vi "TxtHeaderAdvGen.vi"(0 "VarPar":string caption="Param de Balayage Princ", 1 "NomDon":string[](array[string])=["RTêta;", "X&Y;"], 3 "2ndParam":dbl[](array[numeric]) format="%#_15e", 5 "NbCourbe":i32=1 caption="Nb de Balayage", 7 "VarPar Sec":string caption="Param de Balayage Sec", 9 "IndCourbe":i64 caption="Numéro de Balayage", 11 "error in":errorcluster, 12 "Mode":u16(ring) items=["Scan", "Log"], 14 "UnitDon":string[][](array[string])=[["(V)", "(°)"]] caption="Unités Données") -> (4 "Scan list":string[](array[string]), 10 "Entête":string, 15 "error out":errorcluster)   [LabVIEW 2010]
doc: "Ce Vi créer la ligne d'entête du fichier texte de sauvegarde à partir du nombre de courbe voulu."
panel:
  # "Chaque ligne correspond aux différentes unités de \nl'élément correspondant du tableau NomDon. Un élément \"NomDon\" peut avoir plusieurs paramètres (unités) mesurés, mais seulement le premier apparait dans la scanlist. Par contre ils apparaissent tous dans l'entête"
  # ": Chaque item correspond à un élément de plus dans la scan list"
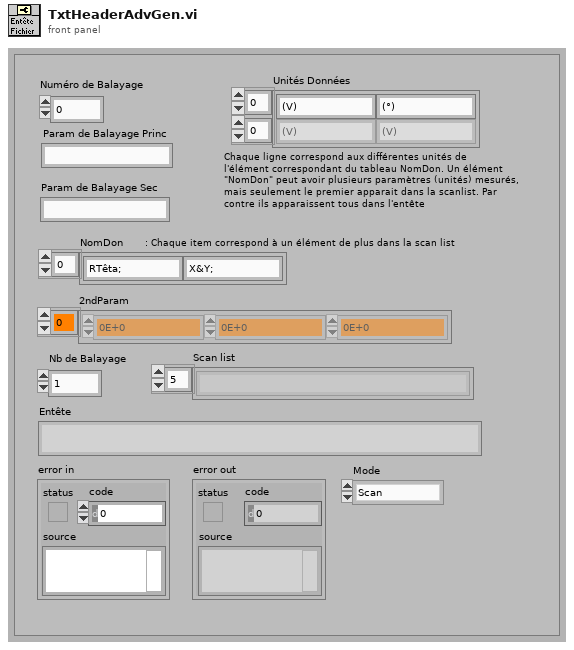
[diagram p1: front panel]
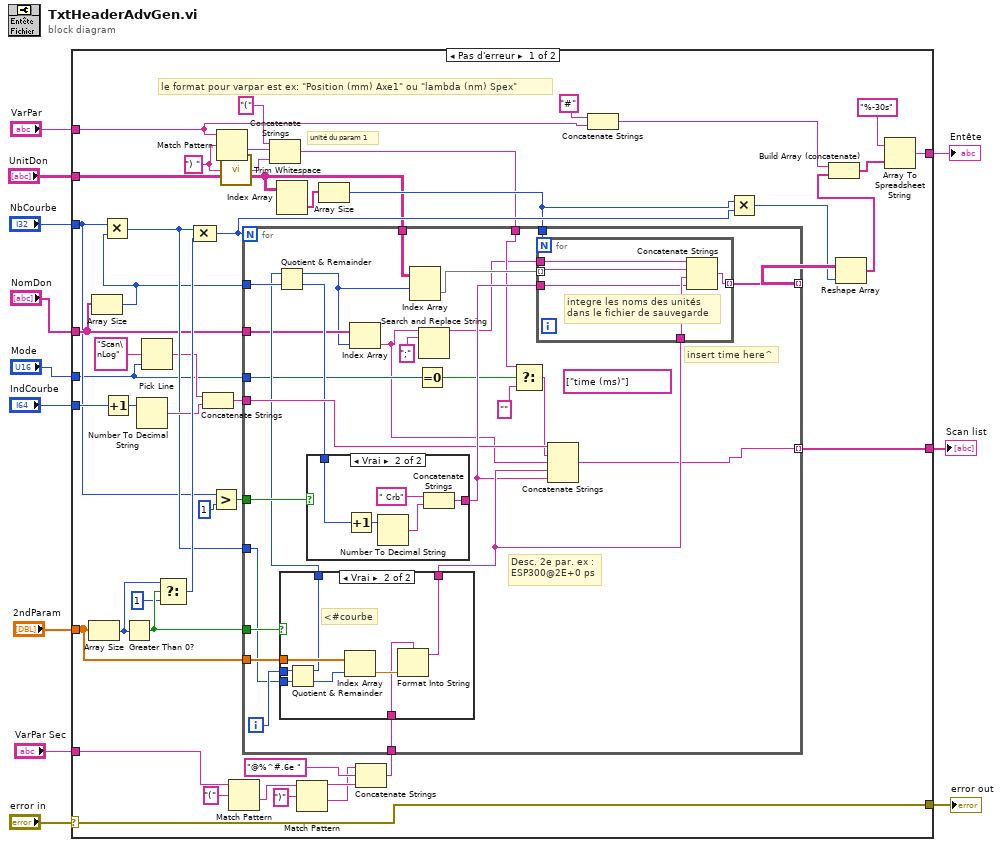
[diagram p0: block diagram]
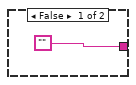
[diagram p2: hidden frame]
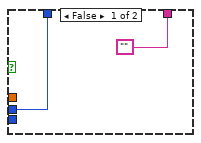
[diagram p3: hidden frame]
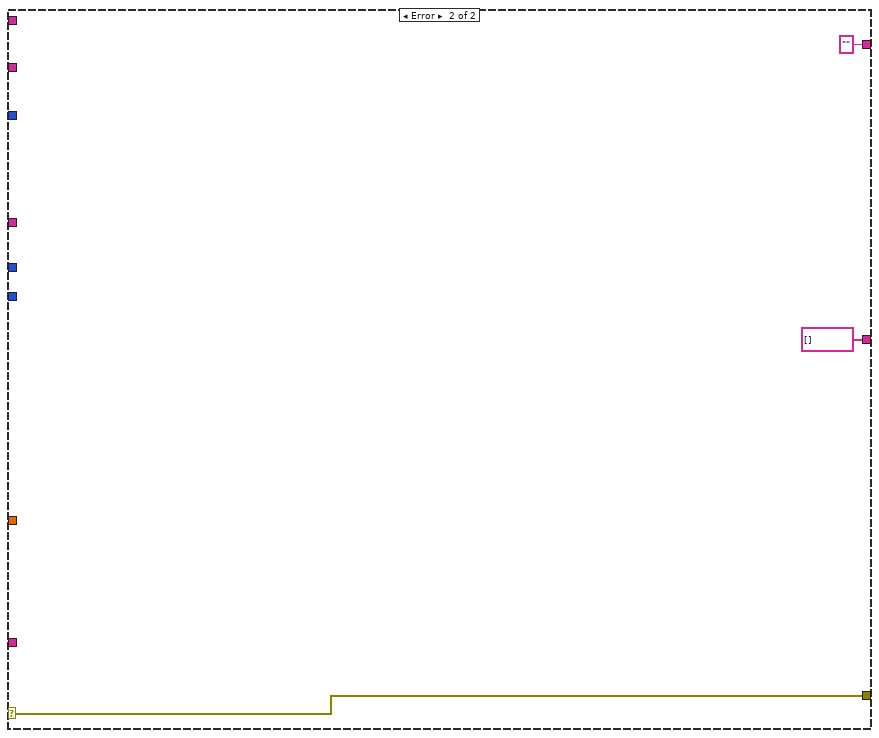
[diagram p4: hidden frame]
diagram:
  n1 = case shown="Pas d'erreur" "error in" {
    selector: "error in" -> [w56 w109]
    tunnel: [w56 w109] -> w11
    tunnel: "NbCourbe" -> [w19 _]
    tunnel: [w29 string[] []] -> w9
    tunnel: [w55 "" ("spreadsheet string")] -> w8
    tunnel: "IndCourbe" -> [w45 _]
    tunnel: "2ndParam" -> [w51 _]
    tunnel: "UnitDon" -> [w27 _]
    tunnel: "NomDon" -> [w25 _]
    tunnel: "VarPar" -> [w15 _]
    tunnel: "VarPar Sec" -> [w23 _]
    tunnel: "Mode" -> [w18 _]
    frame No Error {
      w31 = ") " ("expression régulière")
      # "le format pour varpar est ex: \"Position (mm) Axe1\" ou \"lambda (nm) Spex\""
      # "unité du param 1"
      n2 = Array Size(array=w51) -> (size(s)=w52:i32)
      n3 = Array Size(array=w25) -> (size(s)=w24:i32)
      n4 = Multiply(x=w19, y=w24) -> (x*y=w28:i32)
      n5 = Increment(x=w45) -> (x+1=w44:i64)
      n6 = Greater Than 0?(x=w52) -> (x > 0?=w54:bool)
      n7 = Number To Decimal String(number=w44) -> (decimal integer string=w39:string)  [unwired: 1 in]
      n8 = Pick Line(multi-line string="Scan\nLog", line index=w18) -> (output string=w20:string)  [unwired: 1 in]
      n9 = Select(t=w52, s=w54, f=1 ("NbCourbe")) -> (s? t:f=w46:i32)
      n10 = Compound Arithmetic op=MULTIPLY(w28, w46) -> (w41:i32)
      n11 = Concatenate Strings(w20, w39) -> (w38:string)
      n12 = Greater?(x=w19, y=1) -> (0:w43:bool)
      n13 = Match Pattern(string=w15, regular expression=w31) -> (after substring=w33:string)  [unwired: 1 in, 3 out]
      n14 = call <vilib>:"Trim Whitespace.vi"("string"=w31) -> ("trimmed string"=w30:string)  [unwired: 1 in]
      n15 = Match Pattern(string=w23, regular expression="(" ("expression régulière")) -> (after substring=w36:string)  [unwired: 1 in, 3 out]
      n16 = Concatenate Strings("(" ("expression régulière"), w33, w30) -> (w22:string)
      n17 = Index Array(array=w27) -> (element=w26:string[])  [unwired: 2 in]
      n18 = Match Pattern(string=w36, regular expression=")" ("expression régulière")) -> (before substring=w35:string, after substring=w34:string)  [unwired: 1 in, 2 out]
      n19 = Array Size(array=w26) -> (size(s)=w37:i32)
      n20 = Concatenate Strings(w34, "@%^#.6e ", w35) -> (w48:string)
      n21 = for {
        N: w41 -> [_]
        tunnel: [w63] -> w29 mode=indexing
        tunnel: w22 -> [w68]
        tunnel: w54 -> [w85]
        tunnel: w51 -> [w84]
        tunnel: w48 -> [w83]
        tunnel: w28 -> [w81]
        tunnel: w38 -> [w76]
        tunnel: [w62] -> w17 mode=indexing
        tunnel: w43 -> [w80]
        tunnel: w27 -> [w75]
        tunnel: w37 -> [w79]
        tunnel: w24 -> [w73]
        tunnel: w25 -> [w70]
        tunnel: w18 -> [w67]
        i -> [w82]
        (unwired) string[] ["time (ms)"] ("tableau")
        # "insert time here^"
        # "Desc. 2e par. ex : \nESP300@2E+0 ps"
        n22 = case shown="Vrai" w85 {
          tunnel: ["" w103] -> w78
          tunnel: w84 -> [_ w106]
          tunnel: w82 -> [w97 w102]
          tunnel: w83 -> [_ w104]
          tunnel: w81 -> [_ w101]
          tunnel: [w97 w99] -> w72
          frame False {
          }
          frame True {
            # "<#courbe"
            n23 = Quotient & Remainder(x=w102, y=w101) -> (x-y*floor(x/y)=w99:i32, floor(x/y)=w100:i32)
            n24 = Index Array(array=w106, index=w100) -> (element=w105:dbl)
            n25 = Format Into String(format string=w104, w105) -> (resulting string=w103:string)  [unwired: 2 in, 1 out]
          }
        }
        n26 = Quotient & Remainder(x=w72, y=w73) -> (x-y*floor(x/y)=w69:i32, floor(x/y)=w71:i32)
        n27 = case shown="Vrai" w80 {
          tunnel: ["" w95] -> w77
          tunnel: w71 -> [_ w92]
          frame False {
          }
          frame True {
            n28 = Increment(x=w92) -> (x+1=w96:i32)
            n29 = Number To Decimal String(number=w96) -> (decimal integer string=w94:string)  [unwired: 1 in]
            n30 = Concatenate Strings(" Crb" ("chaîne"), w94) -> (w95:string)
          }
        }
        n31 = Index Array(array=w70, index=w69) -> (element=w59:string)
        n32 = Index Array(array=w75, index (row)=w69) -> (element=w74:string[])  [unwired: 1 in]
        n33 = Equal To 0?(x=w67) -> (x = 0?=w66:bool)
        n34 = Search and Replace String(input string=w59, search string=";" ("chaîne recherchée")) -> (result string=w60:string)  [unwired: 6 in, 3 out]
        n35 = Select(t=w68, s=w66, f="" ("cas faux")) -> (s? t:f=w65:string)
        n36 = for {
          N: w79 -> [_]
          tunnel: w60 -> [w90]
          tunnel: [w87] -> w62 mode=indexing
          tunnel: w74 -> [w86] mode=indexing
          tunnel: w78 -> [w89]
          tunnel: w77 -> [w88]
          # "integre les noms des unités dans le fichier de sauvegarde"
          n37 = Concatenate Strings(w90, w86, w89, w88) -> (w87:string)
        }
        n38 = Concatenate Strings(w76, w65, w59, w78, w77) -> (w63:string)
      }
      n39 = Concatenate Strings("#" ("chaîne"), w15) -> (w13:string)
      n40 = Multiply(x=w37, y=w41) -> (x*y=w16:i32)
      n41 = Reshape Array(w17, w16) -> (w42:string[])
      n42 = Build Array (concatenate)(w13, w42) -> (w58:string[])
      n43 = Array To Spreadsheet String(array=w58, 3:"%-30s" ("format string")) -> (spreadsheet string=w55:string)  [unwired: 1 in]
    }
    frame Error {
    }
  }
  "error out" <- w11
  "Scan list" <- w9
  "Entête" <- w8
